vi "TwWaitForNewData.vi"(2 "WaitForEventReset":bool, 3 "Timeout":i32=100, 4 "TSharedMemoryDesc in":T1, 5 "error in (no error)":errorcluster) -> (0 "TSharedMemoryDesc out":T1, 1 "error out":errorcluster)   [LabVIEW 2009]
uses:
  TSharedMemoryDesc.ctl
  Dblx16.ctl
  charX256.ctl
  charX128.ctl
  TofDaqDll.dll
types:
  T1 = typedef "TSharedMemoryDesc.ctl" = cluster{"NbrSamples":i32, "NbrRawSamples":i32, "NbrPeaks":i32, "NbrWaveforms":i32, "NbrSegments":i32, "NbrBlocks":i32, "NbrMemories":i32, "NbrBufs":i32, "NbrWrites":i32, "NbrRuns":i32, "iWaveform":i32, "iSegment":i32, "iBlock":i32, "iMemory":i32, "iBuf":i32, "iWrite":i32, "iRun":i32, "TotalBufsRecorded":i32, "TotalBufsProcessed":i32, "TotalBufsWritten":i32, "OverallBufsProcessed":i32, "TotalNbrMemories":i32, "TotalMemoriesProcessed":i32, "RawDataRecordedBuf1":u32, "RawDataRecordedBuf2":u32, " RawDataLastElementInBuffer1 ":u32, " RawDataLastElementInBuffer2":u32, "RawDataProcessedBuf1":u32, "RawDataProcessedBuf2":u32, "RawDataWrittenBuf1":u32, "RawDataWrittenBuf2":u32, "SampleInterval":sgl, "TofPeriod":i32, "dummy":i32, "BlockPeriod":i64, "BlockPulseDelay":i64, " BlockDelay ":i64, "SingleIonSignal":sgl, "SingleIonSignal2":sgl, "MassCalibMode":i32, "MassCalibMode2":i32, "NbrMassCalibParams":i32, "NbrMassCalibParams2":i32, "p":T2, "p2":T2, "R0":sgl, "dm":sgl, "m0":sgl, "secondTof":u8, "chIniFileName":T3, "CurrentDataFileName":T3, "dummy":i8, "dummy 2":i8, "dummy 3":i8, "DaqMode":i32, " AcquisitionMode ":i32, "CombineMode":i32, "RecalibFreq":i32, "AcquisitionLogText":T3, " AcquisitionLogTime ":u64, "TimeZero":u64, "ExternalLock":u32, "ProcessingLevel":u32, "AttributeType":i32, "AttributeObject":T3, "AttributeName":T4, " AttributeInt ":i32, " AttributeDouble ":dbl, "EnableVarNbrMemories":u8, "dummy 4":i8, "dummy 5":i8, "dummy 6":i8, " NbrSteps":i32, "  CurrentStepAtBuf ":i32, "NbrMemoriesForCurrentStep":i32}
  T2 = typedef "Dblx16.ctl" = cluster{"0":dbl, "1":dbl, "2":dbl, "3":dbl, "4":dbl, "5":dbl, "6":dbl, "7":dbl, "8":dbl, "9":dbl, "10":dbl, "11":dbl, "12":dbl, "13":dbl, "14":dbl, "15":dbl}
  T3 = typedef "charX256.ctl" = cluster{i8, i8, i8, i8, i8, i8, i8, i8, i8, i8, i8, i8, i8, i8, i8, i8, i8, i8, i8, i8, i8, i8, i8, i8, i8, i8, i8, i8, i8, i8, i8, i8, i8, i8, i8, i8, i8, i8, i8, i8, i8, i8, i8, i8, i8, i8, i8, i8, i8, i8, i8, i8, i8, i8, i8, i8, i8, i8, i8, i8, i8, i8, i8, i8, i8, i8, i8, i8, i8, i8, i8, i8, i8, i8, i8, i8, i8, i8, i8, i8, i8, i8, i8, i8, i8, i8, i8, i8, i8, i8, i8, i8, i8, i8, i8, i8, i8, i8, i8, i8, i8, i8, i8, i8, i8, i8, i8, i8, i8, i8, i8, i8, i8, i8, i8, i8, i8, i8, i8, i8, i8, i8, i8, i8, i8, i8, i8, i8, i8, i8, i8, i8, i8, i8, i8, i8, i8, i8, i8, i8, i8, i8, i8, i8, i8, i8, i8, i8, i8, i8, i8, i8, i8, i8, i8, i8, i8, i8, i8, i8, i8, i8, i8, i8, i8, i8, i8, i8, i8, i8, i8, i8, i8, i8, i8, i8, i8, i8, i8, i8, i8, i8, i8, i8, i8, i8, i8, i8, i8, i8, i8, i8, i8, i8, i8, i8, i8, i8, i8, i8, i8, i8, i8, i8, i8, i8, i8, i8, i8, i8, i8, i8, i8, i8, i8, i8, i8, i8, i8, i8, i8, i8, i8, i8, i8, i8, i8, i8, i8, i8, i8, i8, i8, i8, i8, i8, i8, i8, i8, i8, i8, i8, i8, i8, i8, i8, i8, i8, i8, i8, i8, i8, i8, i8, i8, i8}
  T4 = typedef "charX128.ctl" = cluster{i8, i8, i8, i8, i8, i8, i8, i8, i8, i8, i8, i8, i8, i8, i8, i8, i8, i8, i8, i8, i8, i8, i8, i8, i8, i8, i8, i8, i8, i8, i8, i8, i8, i8, i8, i8, i8, i8, i8, i8, i8, i8, i8, i8, i8, i8, i8, i8, i8, i8, i8, i8, i8, i8, i8, i8, i8, i8, i8, i8, i8, i8, i8, i8, i8, i8, i8, i8, i8, i8, i8, i8, i8, i8, i8, i8, i8, i8, i8, i8, i8, i8, i8, i8, i8, i8, i8, i8, i8, i8, i8, i8, i8, i8, i8, i8, i8, i8, i8, i8, i8, i8, i8, i8, i8, i8, i8, i8, i8, i8, i8, i8, i8, i8, i8, i8, i8, i8, i8, i8, i8, i8, i8, i8, i8, i8, i8, i8}
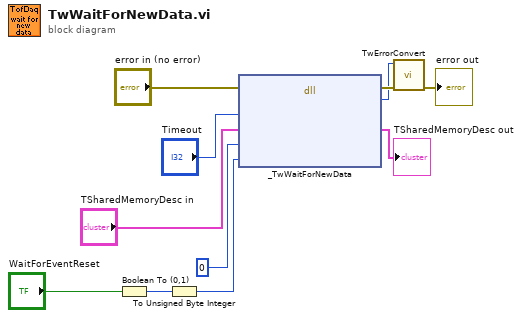
[diagram p0: block diagram]
diagram:
  n1 = Boolean To (0,1)(Boolean="WaitForEventReset") -> (0, 1=w4:i16)
  n2 = To Unsigned Byte Integer(number=w4) -> (unsigned 8bit integer=w3:u8)
  n3 = dll-call lib="C:/src/TofDaq/APIandWrappers/LabView/TofDaqDll/TofDaqDll.dll" fn="_TwWaitForNewData"(error in="error in (no error)", "Timeout"="Timeout", "pBufDesc"="TSharedMemoryDesc in", "pShMem"=u32 0, "WaitForEventReset"=w3) -> (error out=w10:errorcluster, "TwRetVal"=w8:i32, "pBufDesc"=→"TSharedMemoryDesc out":T1)  [unwired: 4 in, 2 out]
  n4 = call "TwErrorConvert.vi"("error in (no error)"=w10, "error code"=w8) -> ("error out"=→"error out":errorcluster)  [unwired: 9 out]
